vi "Measurement Logic.vi"() -> ()   [LabVIEW 2024, in "OneShot-SingleTone.lvlib"]
uses:
  OneShot-SingleTone.lvlib
  <vilib>/Plug-In SDKs/Measurements/Measure Call Context/Measure Call Context.lvclass
  Measurement Configuration.ctl
  Measurement Results.ctl
  <vilib>/addons/_NISVFA/_Generation/Signal Generation/SV Signal/sv_System Timing Model.ctl
  C:/Program Files/NI/LVAddons/nisvt/1/examples/Sound and Vibration/Audio Measurements/subVIs/sv_AO Channel Configuration.ctl
  C:/Program Files/NI/LVAddons/nisvt/1/examples/Sound and Vibration/Audio Measurements/subVIs/sv_AI Channel Configuration.ctl
  <vilib>/addons/_NISVFA/_Generation/Signal Generation/SV Signal/SV Signal.lvclass/SV Signal.ctl
  <vilib>/addons/_NISVFA/_Generation/Signal Generation/SV Signal/Write Synchronization Pulse Parameters.vi
  <vilib>/addons/_NISVFA/_Generation/Signal Generation/SV Signal/Write Profile.vi
  <vilib>/addons/_NISVFA/_Generation/Signal Generation/SV Signal/Write Ramp-Up.vi
  <vilib>/addons/_NISVFA/_Generation/Signal Generation/SV Signal/Write Ramp-Down.vi
  <vilib>/addons/_NISVFA/_Generation/Signal Generation/SV Sinusoid/SV Sinusoid.lvclass
  <vilib>/addons/_NISVFA/_Generation/Signal Generation/SV Sinusoid/Configure Sine.vi
  <vilib>/addons/_NISVFA/_Generation/Signal Generation/SV Signal/Write System Timing Model.vi
  <vilib>/addons/_NISVFA/_Generation/Signal Generation/SV Signal/Write Transition Profile.vi
  <vilib>/addons/_NISVFA/_Generation/Signal Generation/SV Signal/Write Measurement Duration.vi
  <vilib>/addons/_NISVFA/_Generation/Signal Generation/SV Function/Write Measurement Cycles.vi
  <vilib>/addons/_NISVFA/_Generation/Signal Generation/SV Signal/Write Pre-Measurement Settling Duration.vi
  <vilib>/addons/_NISVFA/_Generation/Signal Generation/SV Function/Write Pre-Measurement Settling Cycles.vi
  <extravilib>/ChannelInstances/Event Messenger-bool/Instantiate.vi
  <vilib>/addons/_NISVFA/_Generation/Signal Generation/SV Signal/SV Signal.lvclass
  C:/Program Files/NI/LVAddons/nisvt/1/examples/Sound and Vibration/SoundVib_Audio Examples.lvlib
panel:
  out "measurement results":T1={"band start (Hz) out"=0.0, "band stop (Hz) out"=0.0, "detected frequency (Hz)"=0.0, "detected amplitude"=0.0, "acquired response"=[0.0], "measurement subset"=[0.0], "acquired response t0"=0.0, "acquired response dt"=0.0, "measurement subset t0"=0.0, "measurement subset dt"=0.0, "error"=FALSE, "error code"=0, "error source"="Empty", "THD maximum harmonic out"=9} {"THD maximum harmonic out" min=-1 max=1000; "detected amplitude" format="%.3g"; "band stop (Hz) out" format="%.2f"; "band start (Hz) out" format="%.2f"}
  in  "measurement configuration":T2={"THD maximum harmonic"=1, "measurement duration (s)"=1.2, "measurement cycles"=32.0, "band start (Hz)"=32.0, "band stop (Hz)"=64.0, "ramp up (s)"=64.0, "ramp down (s)"=-32.0, "settle time (s)"=-32.0, "settle cycles"=-64.0, "AI range"=-64.0, "AO range"=1.0, "output channel"="Dev1/ao0", "input channel"="Dev1/ai0", "frequency (Hz)"=1.0, "amplitude"=1.0, "sample rate (Hz)"=0.05} {"sample rate (Hz)" min=0.0 format="%.2p"; "amplitude" format="%.3g"; "frequency (Hz)" format="%.2f"; "AO range" format="±  %.3g"; "settle cycles" min=0.0; "ramp down (s)" min=0.0 format="%.2p"; "band stop (Hz)" format="%.2f"; "measurement cycles" min=1.0; "THD maximum harmonic" min=-1 max=1000}
  out "measure call context out":refnum<class "Measure Call Context.lvclass">
  in  "measure call context in":refnum<class "Measure Call Context.lvclass">
  out "error out":errorcluster
  in  "error in":errorcluster
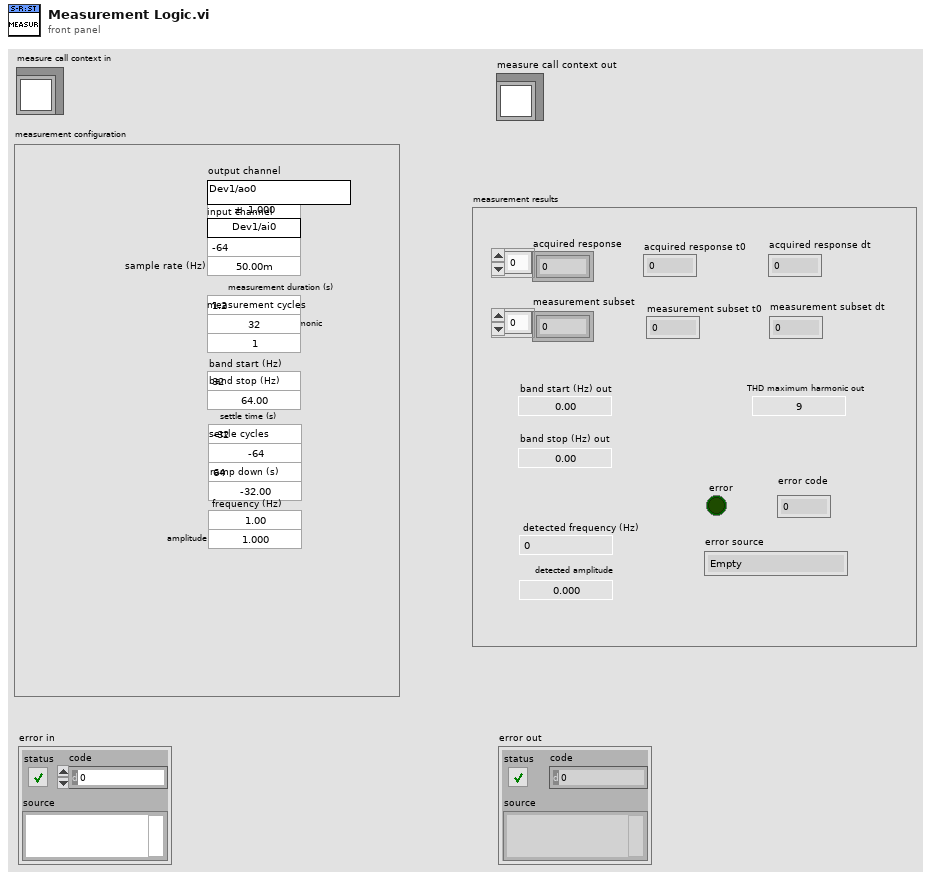
[diagram p1: front panel]
types:
  T1 = typedef "OneShot-SingleTone.lvlib/Measurement Results.ctl" = cluster{"band start (Hz) out":dbl, "band stop (Hz) out":dbl, "detected frequency (Hz)":dbl, "detected amplitude":dbl, "acquired response":dbl[], "measurement subset":dbl[], "acquired response t0":dbl, "acquired response dt":dbl, "measurement subset t0":dbl, "measurement subset dt":dbl, "error":bool, "error code":i32, "error source":string, "THD maximum harmonic out":i32}
  T2 = typedef "OneShot-SingleTone.lvlib/Measurement Configuration.ctl" = cluster{"THD maximum harmonic":i32, "measurement duration (s)":dbl, "measurement cycles":dbl, "band start (Hz)":dbl, "band stop (Hz)":dbl, "ramp up (s)":dbl, "ramp down (s)":dbl, "settle time (s)":dbl, "settle cycles":dbl, "AI range":dbl, "AO range":dbl, "output channel":string, "input channel":string, "frequency (Hz)":dbl, "amplitude":dbl, "sample rate (Hz)":dbl}
  T3 = cluster{"measured (s)":dbl[], "maximum (samples)":i32}
  T4 = typedef "SoundVib_Audio Examples.lvlib/sv_AI Channel Configuration.ctl" = cluster{"DAQmx Channel":tag, "Channel Type":u16, "Max":dbl, "Sensitivity":dbl, "Coupling":enum16{"AC", "DC"}, "excitation":enum16{"Off", "Min", "Max"}, "input terminal configuration":i32}
  T5 = typedef "SoundVib_Audio Examples.lvlib/sv_AO Channel Configuration.ctl" = cluster{"DAQmx Channel":tag, "Max":dbl, "output terminal configuration":i32}
  T6 = cluster{"enable leading":bool, "enable trailing":bool, "duration [s]":dbl, "type":enum16{"Noise", "MLS", "Chirp", "Monopulse", "Custom"}, "level":dbl}
  T7 = typedef "SV Signal.lvclass/sv_System Timing Model.ctl" = i64
  T8 = typedef "Event Messenger-bool.lvlib/))Channel.ctl" = refnum<queue>
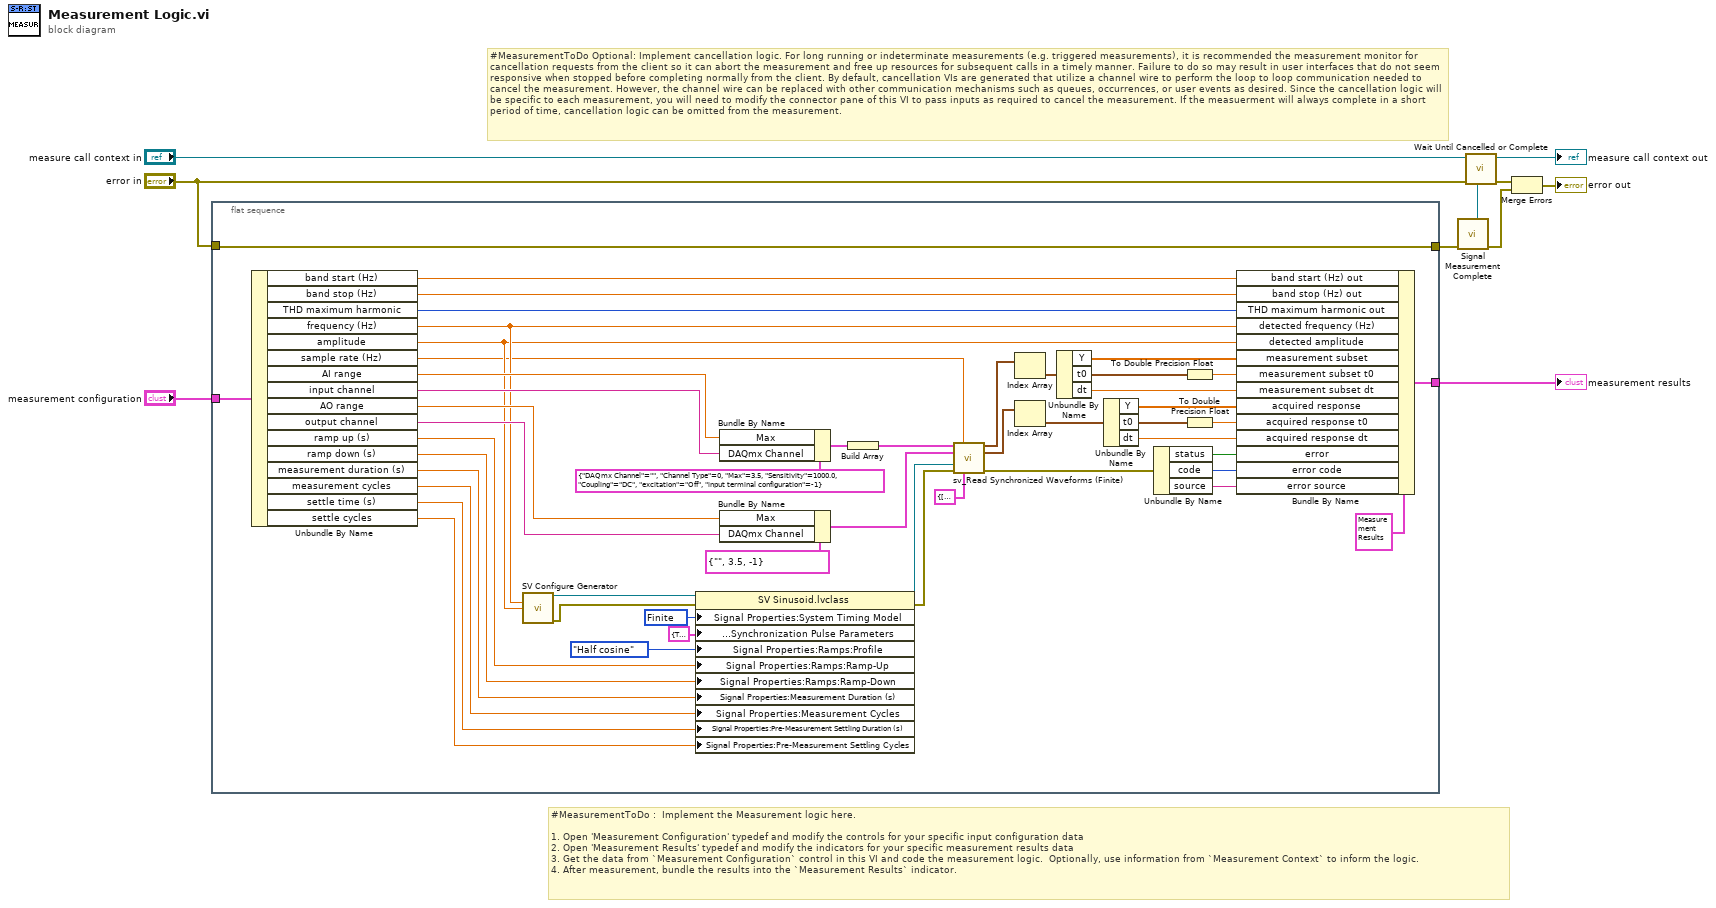
[diagram p0: block diagram]
diagram:
  # "#MeasurementToDo Optional: Implement cancellation logic. For long running or indeterminate measurements (e.g. triggered measurements), it is recommended the measurement monitor for cancellation requests from the client so it can abort the measurement and free up resources for subsequent calls in a timely manner. Failure to do so may result in user interfaces that do not seem responsive when stopped before completing normally from the client. By default, cancellation VIs are generated that utilize a channel wire to perform the loop to loop communication needed to cancel the measurement. However, the channel wire can be replaced with other communication mechanisms such as queues, occurrences, or user events as desired. Since the cancellation logic will be specific to each measurement, you will need to modify the connector pane of this VI to pass inputs as required to cancel the measurement. If the measuerment will always complete in a short period of time, cancellation logic can be omitted from the measurement."
  # "#MeasurementToDo :  Implement the Measurement logic here.\n\n1. Open 'Measurement Configuration' typedef and modify the controls for your specific input configuration data\n2. Open 'Measurement Results' typedef and modify the indicators for your specific measurement results data\n3. Get the data from `Measurement Configuration` control in this VI and code the measurement logic.  Optionally, use information from `Measurement Context` to inform the logic.\n4. After measurement, bundle the results into the `Measurement Results` indicator."
  n1 = flat-sequence {
    tunnel: "measurement configuration" -> [w56]
    tunnel: [w58] -> w9
    tunnel: "error in" -> [w57]
    tunnel: [w57] -> w5
    frame #0 {
      w52 = T7 10178 items=["Finite"=10178, "-"=-1, "Continuous"=10123, "-"=-2, "Settled"=110123, "Averaged"=210123, "Discrete Sweep"=310123, "Continuous Sweep"=410123] ("System Timing Model")
      n2 = Unbundle By Name(w56) -> ("band start (Hz)"=w55:dbl, "band stop (Hz)"=w54:dbl, "THD maximum harmonic"=w53:i32, "frequency (Hz)"=w36:dbl, "amplitude"=w35:dbl, "sample rate (Hz)"=w12:dbl, "AI range"=w40:dbl, "input channel"=w39:string, "AO range"=w38:dbl, "output channel"=w37:string, "ramp up (s)"=w34:dbl, "ramp down (s)"=w33:dbl, "measurement duration (s)"=w32:dbl, "measurement cycles"=w31:dbl, "settle time (s)"=w30:dbl, "settle cycles"=w29:dbl)
      n3 = call-poly <vilib>:"SV Configure Generator.vi"("frequency (Hz)"=w36, "amplitude"=w35) -> ("signal configuration"=w51:refnum<class "SV Sinusoid.lvclass">, "error out"=w47:errorcluster)  [unwired: 12 in]
      n4 = property class="SV Sinusoid.lvclass"(reference=w51, error in=w47, "Signal Properties:System Timing Model"=w52, "Signal Properties:Synchronization Pulses:Synchronization Pulse Parameters"=T6 {"enable leading"=TRUE, "enable trailing"=FALSE, "duration [s]"=0.005, "type"=enum."Noise", "level"=0.5} ("Synchronization Pulses:All Elements"), "Signal Properties:Ramps:Profile"=enum16{"Linear", "Half cosine"}."Half cosine" ("Ramp Parameters:Profile"), "Signal Properties:Ramps:Ramp-Up"=w34, "Signal Properties:Ramps:Ramp-Down"=w33, "Signal Properties:Measurement Duration (s)"=w32, "Signal Properties:Measurement Cycles"=w31, "Signal Properties:Pre-Measurement Settling Duration (s)"=w30, "Signal Properties:Pre-Measurement Settling Cycles"=w29) -> (reference out=w48:refnum<class "SV Sinusoid.lvclass">, error out=w49:errorcluster)
      n5 = Bundle By Name(cluster=T4 {"DAQmx Channel"="", "Channel Type"=0, "Max"=3.5, "Sensitivity"=1000.0, "Coupling"=enum."DC", "excitation"=enum."Off", "input terminal configuration"=-1} ("Channel Information"), "Max"=w40, "DAQmx Channel"=w39) -> (w44:T4)
      n6 = Bundle By Name(cluster=T5 {"DAQmx Channel"="", "Max"=3.5, "output terminal configuration"=-1} ("analog output channel"), "Max"=w38, "DAQmx Channel"=w37) -> (w42:T5)
      n7 = Build Array(w44) -> (w43:T4[])
      n8 = call "sv_Read Synchronized Waveforms (Finite).vi"("analog input channels"=w43, "sample rate (Hz)"=w12, "analog output channel"=w42, "signal configuration in"=w48, "error in (no error)"=w49, "propagation delay"=T3 {"measured (s)"=[], "maximum (samples)"=200}) -> ("waveforms to measure"=w28:waveform(dbl)[], "full waveforms"=w25:waveform(dbl)[], "error out"=w24:errorcluster)  [unwired: 5 in, 2 out]
      n9 = Index Array(array=w28) -> (element=w27:waveform(dbl))  [unwired: 1 in]
      n10 = Index Array(array=w25) -> (element=w26:waveform(dbl))  [unwired: 1 in]
      n11 = Unbundle By Name(w27) -> ("Y"=w22:dbl[], "t0"=w21:timestamp, "dt"=w19:dbl)
      n12 = Unbundle By Name(w26) -> ("Y"=w18:dbl[], "t0"=w16:timestamp, "dt"=w17:dbl)
      n13 = Unbundle By Name(w24) -> ("status"=w23:bool, "code"=w14:i32, "source"=w13:string)
      n14 = To Double Precision Float(number=w21) -> (double precision float=w20:dbl)
      n15 = To Double Precision Float(number=w16) -> (double precision float=w15:dbl)
      n16 = Bundle By Name(cluster=T1 {"band start (Hz) out"=0.0, "band stop (Hz) out"=0.0, "detected frequency (Hz)"=0.0, "detected amplitude"=0.0, "acquired response"=[], "measurement subset"=[], "acquired response t0"=0.0, "acquired response dt"=0.0, "measurement subset t0"=0.0, "measurement subset dt"=0.0, "error"=FALSE, "error code"=0, "error source"="Empty", "THD maximum harmonic out"=9} ("Measurement Results"), "band start (Hz) out"=w55, "band stop (Hz) out"=w54, "THD maximum harmonic out"=w53, "detected frequency (Hz)"=w36, "detected amplitude"=w35, "measurement subset"=w22, "measurement subset t0"=w20, "measurement subset dt"=w19, "acquired response"=w18, "acquired response t0"=w15, "acquired response dt"=w17, "error"=w23, "error code"=w14, "error source"=w13) -> (w58:T1)
    }
  }
  n17 = call "Signal Measurement Complete.vi"("error in (no error)"=w5) -> ("error out"=w3:errorcluster, "done channel"=w4:T8)  [unwired: 9 in]
  n18 = call "Wait Until Cancelled or Complete.vi"("done channel"=w4, "error in (no error)"="error in", "measure call context in"="measure call context in") -> ("error out"=w2:errorcluster, "measure call context out"=→"measure call context out":refnum<class "Measure Call Context.lvclass">)  [unwired: 7 in]
  n19 = Merge Errors(w2, w3) -> (→"error out":errorcluster)
  "measurement results" <- w9
